vi "User Manual Example 3.vi"() -> ()   [LabVIEW 2013]
uses:
  <instrlib>/SRS SR400/Public/Typedefs/Counter.ctl
  <instrlib>/SRS SR400/Public/Typedefs/Counter Input.ctl
  <instrlib>/SRS SR400/Public/Typedefs/Gate Mode.ctl
  <instrlib>/SRS SR400/Public/Typedefs/Discriminator Slope.ctl
  <instrlib>/SRS SR400/Examples/Typedefs/Example 3 Program State.ctl
  <instrlib>/SRS SR400/Public/Typedefs/Menu Display Line.ctl
  <instrlib>/SRS SR400/Public/Typedefs/Status Bit.ctl
  <instrlib>/SRS SR400/SRS SR400.lvlib
panel:
  in  "Discriminator Slope":T1
  in  "Discriminator Level":dbl=0.15
  out "Counts":i16[](array[numeric])
  in  "Gate Width":dbl=0.5
  in  "Gate Delay":dbl=0.3
  in  "Gate Mode":T2=enum."Fixed"
  in  "Dwell Time":dbl
  in  "Number of Periods":u16=10 max=2000 step=1
  in  "Counter Preset":u64=9000000 format="%.0e"
  in  "Counter Input":T3
  in  "Counter":T4=enum."T"
  in  "SRS SR400":refnum<visa-resource-name>
  # "LEVEL Settings"
  # "A GATE Settings"
  # "MODE Settings"
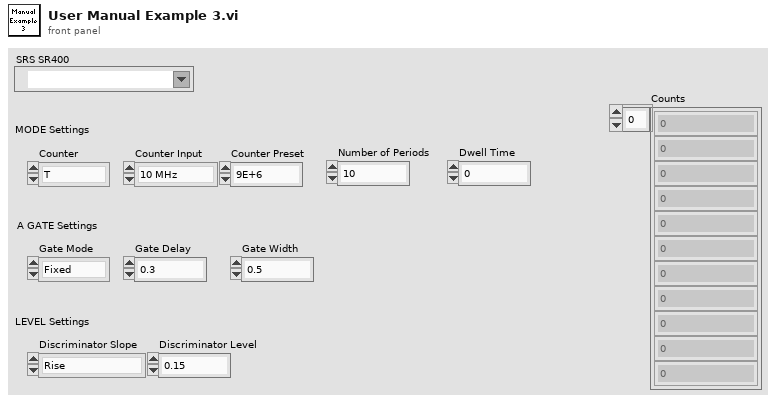
[diagram p1: front panel]
types:
  T1 = typedef "SRS SR400.lvlib/Discriminator Slope.ctl" = enum16{"Rise", "Fall"}
  T2 = typedef "SRS SR400.lvlib/Gate Mode.ctl" = enum16{"CW", "Fixed", "Scan"}
  T3 = typedef "SRS SR400.lvlib/Counter Input.ctl" = enum16{"10 MHz", "INPUT 1", "INPUT 2", "TRIG"}
  T4 = typedef "SRS SR400.lvlib/Counter.ctl" = enum16{"A", "B", "T"}
  T5 = typedef "Example 3 Program State.ctl" = enum16{"Initialize", "Set Scan Parameters", "Reset Count", "Start Count", "Check for Scan Finished", "Check for Data Ready", "Read Counts", "Close Hardware"}
  T6 = typedef "SRS SR400.lvlib/Menu Display Line.ctl" = enum16{"1,1     COUNT", "1,2     A", "1,3     B", "1,4     T", "1,5     N PERIODS", "1,6     AT N", "1,7     D/A OUT", "1,8     D/A RANGE", "1,9     DISPLAY", "2,1     A GATE", "2,2     A DELAY", "2,3     A WIDTH", "3,1     B GATE", "3,2     B DELAY", "3,3     B WIDTH", "4,1     TRIG SLOPE", "4,2     TRIG LVL", "4,3     A DISC SLOPE", "4,4     A DISC MODE", "4,5     A DISC LVL", "4,6     B DISC SLOPE", "4,7     B DISC MODE", "4,8     B DISC LVL", "4,9     T DISC SLOPE", "4,10   T DISC MODE", "4,11   T DISC LVL", "4,12   PORT1 MODE", "4,13   PORT1 LVL", "4,14   PORT2 MODE", "4,15   PORT2 LVL", "5,1     GPIB ADDR", "5,2     RS-232 BAUD", "5,3     RS-232 BITS", "5,4     RS-232 PARITY", "5,5     RS-232 WAIT", "5,6     RS-232 ECHO", "5,7     DATA", "6,1     LCD CONTRAST", "6,2     STORE", "6,3     RECALL"}
  T7 = typedef "SRS SR400.lvlib/Status Bit.ctl" = enum16{"Parameter Changed", "Data Ready", "Scan Finished", "Counter Overrun", "Rate Error", "Recall Error", "SRQ", "Command Error"}
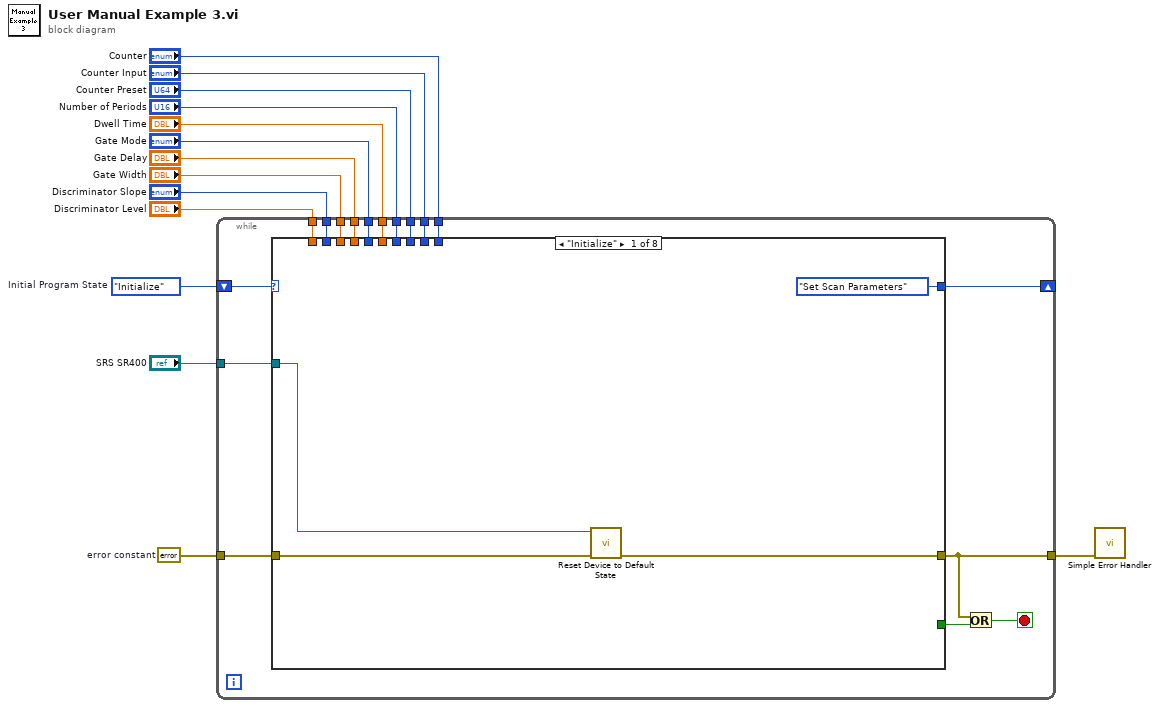
[diagram p0: block diagram]
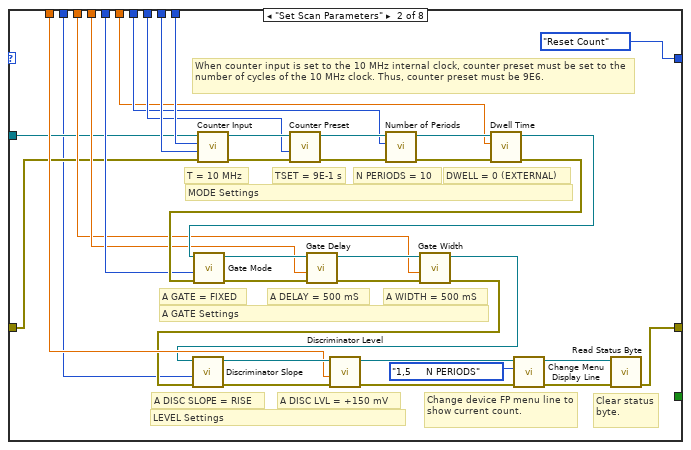
[diagram p2: hidden frame]
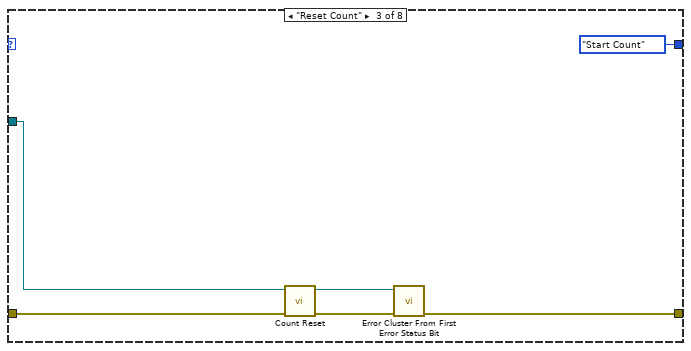
[diagram p3: hidden frame]
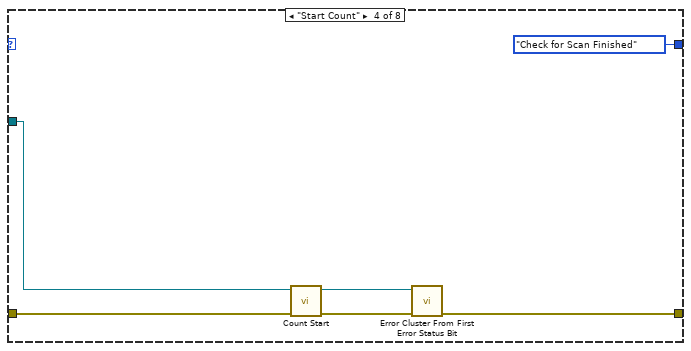
[diagram p4: hidden frame]
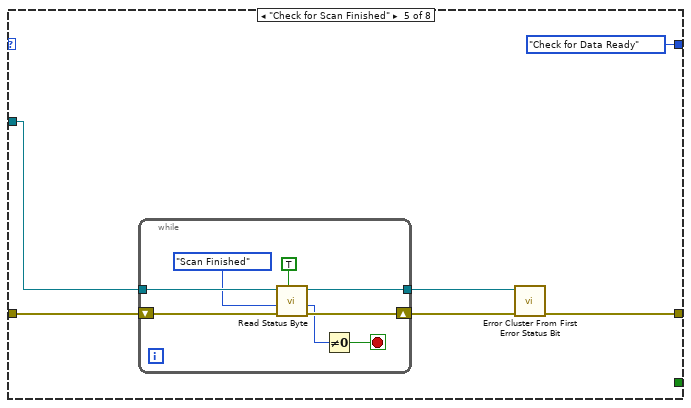
[diagram p5: hidden frame]
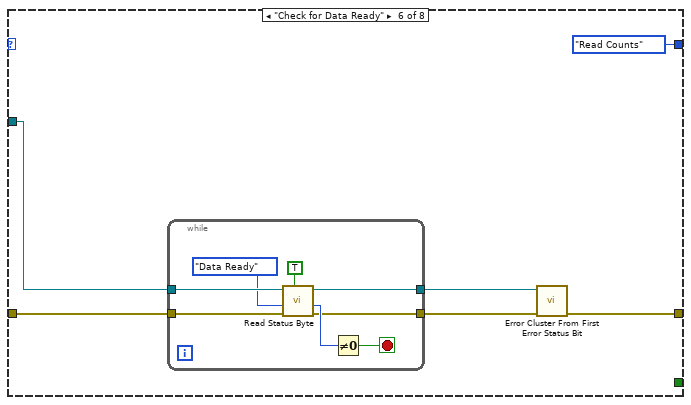
[diagram p6: hidden frame]
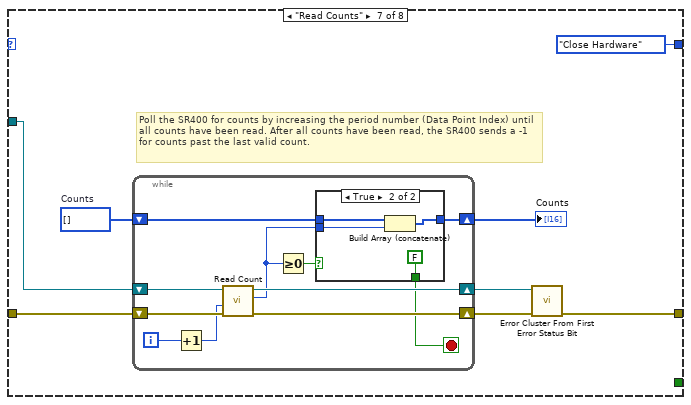
[diagram p7: hidden frame]
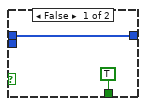
[diagram p8: hidden frame]
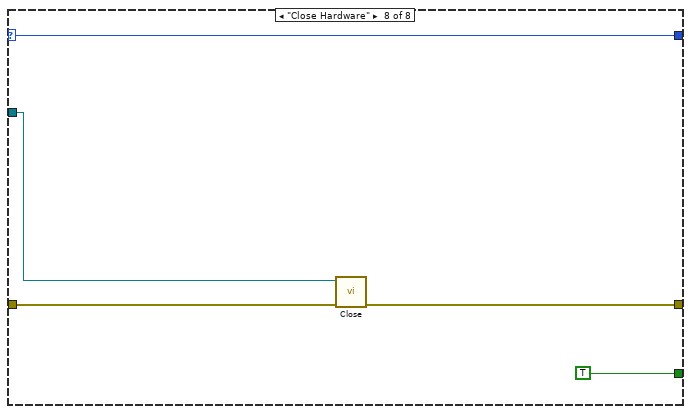
[diagram p9: hidden frame]
diagram:
  w13 = Example_3_Program_State."Initialize"  # Initial Program State
  w14 = errorcluster {"status"=FALSE, "code"=0, "source"=""}  # error constant
  n1 = while {
    tunnel: w14 -> [w31]
    tunnel: "SRS SR400" -> [w29]
    shift-right: [w17] -> _
    shift-left: w13 -> [w30]
    tunnel: "Counter" -> [w26]
    tunnel: "Counter Input" -> [w25]
    tunnel: "Counter Preset" -> [w24]
    tunnel: "Number of Periods" -> [w23]
    tunnel: "Dwell Time" -> [w22]
    tunnel: "Gate Mode" -> [w21]
    tunnel: "Gate Delay" -> [w20]
    tunnel: "Gate Width" -> [w19]
    tunnel: "Discriminator Level" -> [w18]
    tunnel: [w16] -> w2
    tunnel: "Discriminator Slope" -> [w15]
    stop <- w28 stop-if-true
    n2 = case shown="\"Initialize\"" w30 {
      selector: w30 -> [_ _ _ _ _ _ _ w136]
      tunnel: w31 -> [w35 w45 w75 w82 w88 w102 w118 w139]
      tunnel: w29 -> [w34 w46 w76 w81 w87 w101 w117 w138]
      tunnel: [w33 w39 w72 w78 w84 w100 w115 w137] -> w16
      tunnel: [_ _ _ _ _ _ _ TRUE] -> w27
      tunnel: w26 -> [_ w55 _ _ _ _ _ _]
      tunnel: w25 -> [_ w54 _ _ _ _ _ _]
      tunnel: w24 -> [_ w53 _ _ _ _ _ _]
      tunnel: w23 -> [_ w52 _ _ _ _ _ _]
      tunnel: w22 -> [_ w51 _ _ _ _ _ _]
      tunnel: w21 -> [_ w50 _ _ _ _ _ _]
      tunnel: w20 -> [_ w49 _ _ _ _ _ _]
      tunnel: w19 -> [_ w48 _ _ _ _ _ _]
      tunnel: w18 -> [_ w47 _ _ _ _ _ _]
      tunnel: [Example_3_Program_State."Set Scan Parameters" ("Initial Program State") Example_3_Program_State."Reset Count" ("Initial Program State") Example_3_Program_State."Start Count" ("Initial Program State") Example_3_Program_State."Check for Scan Finished" ("Initial Program State") Example_3_Program_State."Check for Data Ready" ("Initial Program State") Example_3_Program_State."Read Counts" ("Initial Program State") Example_3_Program_State."Close Hardware" ("Initial Program State") w136] -> w17
      tunnel: w15 -> [_ w37 _ _ _ _ _ _]
      frame "Initialize" {
        n3 = call <instrlib>:"Reset Device to Default State.vi"("error in (no error)"=w35, "VISA resource name"=w34) -> ("error out"=w33:errorcluster)  [unwired: 8 in, 1 out]
      }
      frame "Set Scan Parameters" {
        # "When counter input is set to the 10 MHz internal clock, counter preset must be set to the number of cycles of the 10 MHz clock. Thus, counter preset must be 9E6."
        # "Clear status byte."
        # "Change device FP menu line to show current count."
        # "DWELL = 0 (EXTERNAL)"
        # "N PERIODS = 10"
        # "LEVEL Settings"
        # "A DISC LVL = +150 mV"
        # "A GATE Settings"
        # "MODE Settings"
        # "A DISC SLOPE = RISE"
        # "A WIDTH = 500 mS"
        # "A DELAY = 500 mS"
        # "A GATE = FIXED"
        # "TSET = 9E-1 s"
        # "T = 10 MHz"
        n4 = call <instrlib>:"Counter Input.vi"("error in (no error)"=w45, "Counter Input (INPUT 1)"=w54, "Counter (A)"=w55, "VISA resource name"=w46) -> ("error out"=w63:errorcluster, "VISA resource name out"=w57:refnum<visa-resource-name>)  [unwired: 5 in, 1 out]
        n5 = call <instrlib>:"Counter Preset.vi"("error in (no error)"=w63, "Counter Preset (1)"=w53, "VISA resource name"=w57) -> ("error out"=w64:errorcluster, "VISA resource name out"=w58:refnum<visa-resource-name>)  [unwired: 6 in, 1 out]
        n6 = call <instrlib>:"Number of Periods.vi"("error in (no error)"=w64, "Number of Periods (1)"=w52, "VISA resource name"=w58) -> ("error out"=w65:errorcluster, "VISA resource name out"=w59:refnum<visa-resource-name>)  [unwired: 6 in, 1 out]
        n7 = call <instrlib>:"Dwell Time.vi"("error in (no error)"=w65, "Dwell Time (1E0 s)"=w51, "VISA resource name"=w59) -> ("error out"=w70:errorcluster, "VISA resource name out"=w69:refnum<visa-resource-name>)  [unwired: 6 in, 1 out]
        n8 = call <instrlib>:"Gate Mode.vi"("error in (no error)"=w70, "Gate Mode (CW)"=w50, "VISA resource name"=w69) -> ("error out"=w66:errorcluster, "VISA resource name out"=w60:refnum<visa-resource-name>)  [unwired: 6 in, 1 out]
        n9 = call <instrlib>:"Gate Delay.vi"("error in (no error)"=w66, "Gate Delay (0.000E-6 s)"=w49, "VISA resource name"=w60) -> ("error out"=w67:errorcluster, "VISA resource name out"=w61:refnum<visa-resource-name>)  [unwired: 6 in, 1 out]
        n10 = call <instrlib>:"Gate Width.vi"("error in (no error)"=w67, "Gate Width (0.005E-6 s)"=w48, "VISA resource name"=w61) -> ("error out"=w42:errorcluster, "VISA resource name out"=w41:refnum<visa-resource-name>)  [unwired: 6 in, 1 out]
        n11 = call <instrlib>:"Discriminator Slope.vi"("error in (no error)"=w42, "Discriminator Slope (Fall)"=w37, "VISA resource name"=w41) -> ("error out"=w68:errorcluster, "VISA resource name out"=w62:refnum<visa-resource-name>)  [unwired: 6 in, 1 out]
        n12 = call <instrlib>:"Discriminator Level.vi"("error in (no error)"=w68, "Discriminator Level (-0.0100 V)"=w47, "VISA resource name"=w62) -> ("error out"=w44:errorcluster, "VISA resource name out"=w43:refnum<visa-resource-name>)  [unwired: 6 in, 1 out]
        n13 = call <instrlib>:"Change Menu Display Line.vi"("error in (no error)"=w44, "Menu Display Line [Menu,Line] (COUNT)"=Menu_Display_Line."1,5     N PERIODS", "VISA resource name"=w43) -> ("error out"=w40:errorcluster, "VISA resource name out"=w38:refnum<visa-resource-name>)  [unwired: 7 in]
        n14 = call <instrlib>:"Read Status Byte.vi"("error in (no error)"=w40, "VISA resource name"=w38) -> ("error out"=w39:errorcluster)  [unwired: 6 in, 3 out]
      }
      frame "Reset Count" {
        n15 = call <instrlib>:"Count Reset.vi"("error in (no error)"=w75, "VISA resource name"=w76) -> ("error out"=w74:errorcluster, "VISA resource name out"=w73:refnum<visa-resource-name>)  [unwired: 8 in]
        n16 = call <instrlib>:"Error Cluster From First Error Status Bit.vi"("error in (no error)"=w74, "VISA resource name"=w73) -> ("error out"=w72:errorcluster)  [unwired: 8 in, 1 out]
      }
      frame "Start Count" {
        n17 = call <instrlib>:"Count Start.vi"("error in (no error)"=w82, "VISA resource name"=w81) -> ("error out"=w80:errorcluster, "VISA resource name out"=w79:refnum<visa-resource-name>)  [unwired: 8 in]
        n18 = call <instrlib>:"Error Cluster From First Error Status Bit.vi"("error in (no error)"=w80, "VISA resource name"=w79) -> ("error out"=w78:errorcluster)  [unwired: 8 in, 1 out]
      }
      frame "Check for Scan Finished" {
        n19 = while {
          tunnel: w87 -> [w94]
          shift-right: [w95] -> w85
          shift-left: w88 -> [w96]
          tunnel: [w89] -> w86
          stop <- w90 stop-if-true
          n20 = call <instrlib>:"Read Status Byte.vi"("Read Status Bit? (F)"=TRUE, "error in (no error)"=w96, "Status Bit (Scan Finished)"=Status_Bit."Scan Finished", "VISA resource name"=w94) -> ("error out"=w95:errorcluster, "Status Bit"=w91:u8, "VISA resource name out"=w89:refnum<visa-resource-name>)  [unwired: 4 in, 1 out]
          n21 = Not Equal To 0?(x=w91) -> (x != 0?=w90:bool)
        }
        n22 = call <instrlib>:"Error Cluster From First Error Status Bit.vi"("error in (no error)"=w85, "VISA resource name"=w86) -> ("error out"=w84:errorcluster)  [unwired: 8 in, 1 out]
      }
      frame "Check for Data Ready" {
        n23 = while {
          tunnel: w101 -> [w109]
          tunnel: w102 -> [w110]
          tunnel: [w104] -> w97
          tunnel: [w105] -> w98
          stop <- w103 stop-if-true
          n24 = call <instrlib>:"Read Status Byte.vi"("Read Status Bit? (F)"=TRUE, "error in (no error)"=w110, "Status Bit (Scan Finished)"=Status_Bit."Data Ready", "VISA resource name"=w109) -> ("error out"=w104:errorcluster, "Status Bit"=w107:u8, "VISA resource name out"=w105:refnum<visa-resource-name>)  [unwired: 4 in, 1 out]
          n25 = Not Equal To 0?(x=w107) -> (x != 0?=w103:bool)
        }
        n26 = call <instrlib>:"Error Cluster From First Error Status Bit.vi"("error in (no error)"=w97, "VISA resource name"=w98) -> ("error out"=w100:errorcluster)  [unwired: 8 in, 1 out]
      }
      frame "Read Counts" {
        w112 = i16[] []  # Counts
        # "Poll the SR400 for counts by increasing the period number (Data Point Index) until all counts have been read. After all counts have been read, the SR400 sends a -1 for counts past the last valid count."
        n27 = while {
          shift-right: [w127] -> w116
          shift-left: w118 -> [w129]
          shift-right: [w126] -> w114
          shift-left: w117 -> [w128]
          shift-right: [w119] -> w111
          shift-left: w112 -> [w120]
          i -> [w125]
          stop <- w121 stop-if-true
          n28 = Increment(x=w125) -> (x+1=w124:i32)
          n29 = call <instrlib>:"Read Count.vi"("error in (no error)"=w129, "Data Point Index (0: Last)"=w124, "VISA resource name"=w128) -> ("error out"=w127:errorcluster, "Count"=w122:i16, "VISA resource name out"=w126:refnum<visa-resource-name>)  [unwired: 6 in]
          n30 = Greater Or Equal To 0?(x=w122) -> (x >= 0?=w123:bool)
          n31 = case shown="True" w123 {
            tunnel: w122 -> [_ w132]
            tunnel: [TRUE FALSE] -> w121
            tunnel: w120 -> [w130 w134]
            tunnel: [w130 w133] -> w119
            frame False {
            }
            frame True {
              n32 = Build Array (concatenate)(w134, w132) -> (w133:i16[])
            }
          }
        }
        "Counts" <- w111
        n33 = call <instrlib>:"Error Cluster From First Error Status Bit.vi"("error in (no error)"=w116, "VISA resource name"=w114) -> ("error out"=w115:errorcluster)  [unwired: 8 in, 1 out]
      }
      frame "Close Hardware" {
        n34 = call <instrlib>:"Close.vi"("error in (no error)"=w139, "VISA resource name"=w138) -> ("error out"=w137:errorcluster)  [unwired: 9 in]
      }
    }
    n35 = Or(x=w16, y=w27) -> (x .or. y?=w28:bool)
  }
  n36 = call <vilib>:"Simple Error Handler.vi"("error in (no error)"=w2) -> ()  [unwired: 4 in, 5 out]
